vi "create file csv.vi"(11 "filename":string) -> (2 "function return":u32, 3 "filename out":string)   [LabVIEW 2019, in "apdm.lvlib"]
doc: "APDM_EXPORT apdm_csv_t apdm_create_file_csv(char *filename);"
uses:
  apdm.lvlib
  Lee Lab/CP FES Walking 2018/Code/Working/LabVIEW/apdm.dll
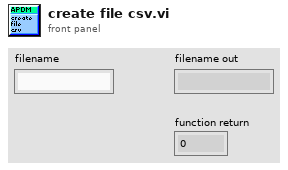
[diagram p1: front panel]
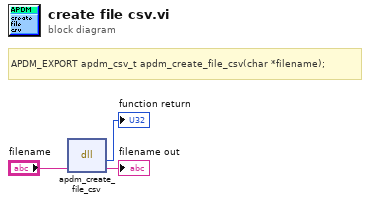
[diagram p0: block diagram]
diagram:
  # "APDM_EXPORT apdm_csv_t apdm_create_file_csv(char *filename);"
  n1 = dll-call lib="C:/Users/jfalesi/Dropbox/Lee Lab/CP FES Walking 2018/Code/Working/LabVIEW/apdm.*" fn="apdm_create_file_csv"("filename"="filename") -> (→"function return":u32, "filename"=→"filename out":string)  [unwired: 3 in, 2 out]
